vi "ASI_serialRelativeMove setpoint.vi"(2 "VISA resource name":refnum<visa-resource-name>="COM7", 3 "error in (no error)":errorcluster, 4 "setpoint":i32, 5 "Axis":string) -> (0 "error out":errorcluster)   [LabVIEW 2015]
doc: "Establishes connection with configured port (default = COM1).\nSends command MOVE X=x Y=y where x and y are integers denoting 10ths of a micron.\nSub-VI SerialWaitForStatusN.vi polls controller with STATUS command until 'N' (not busy) status is returned, or until a configured maximum number of unsuccessful tries (default = 400).\nDisconnects from configured port."
uses:
  <vilib>/Instr/_visa.llb/VISA Flush IO Buffer Mask.ctl
  Instance           1 20Saved   SerialMoveXY .vi
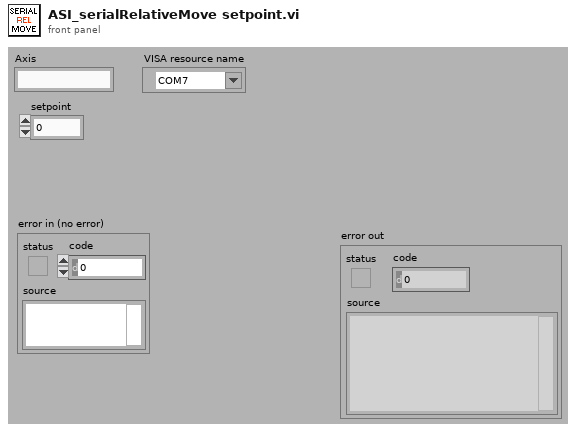
[diagram p1: front panel]
types:
  T1 = typedef "VISA Flush IO Buffer Mask.ctl" = u16
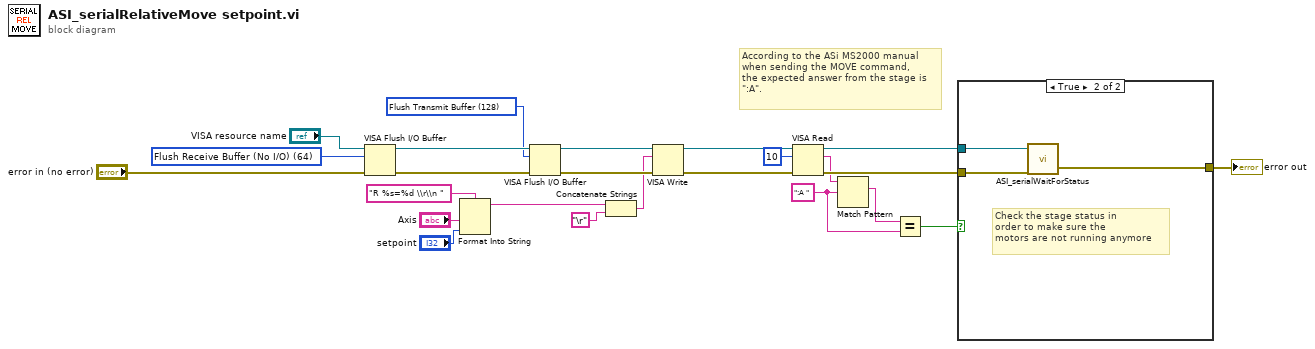
[diagram p0: block diagram]
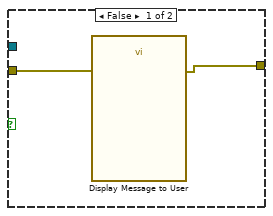
[diagram p2: hidden frame]
diagram:
  w12 = T1 128 items=["Flush Receive Buffer"=16, "Write Transmit Buffer to Device"=32, "Flush Receive Buffer (No I/O)"=64, "Flush Transmit Buffer"=128] ("Mask")
  w15 = T1 64 items=["Flush Receive Buffer"=16, "Write Transmit Buffer to Device"=32, "Flush Receive Buffer (No I/O)"=64, "Flush Transmit Buffer"=128] ("Mask")
  w1 = ":A " ("y")
  # "According to the ASi MS2000 manual\nwhen sending the MOVE command, \nthe expected answer from the stage is\n\":A\"."
  n1 = VISA Flush I/O Buffer(VISA resource name="VISA resource name", mask (16)=w15, error in (no error)="error in (no error)") -> (VISA resource name out=w13:refnum<visa-resource-name>, error out=w14:errorcluster)
  n2 = Format Into String "Format Into String"(format string="R %s=%d \\r\\n ", "Axis", "setpoint") -> (resulting string=w6:string)  [unwired: 2 in, 1 out]
  n3 = VISA Flush I/O Buffer(VISA resource name=w13, mask (16)=w12, error in (no error)=w14) -> (VISA resource name out=w10:refnum<visa-resource-name>, error out=w11:errorcluster)
  n4 = Concatenate Strings(w6, "\r") -> (w4:string)
  n5 = VISA Write(VISA resource name=w10, write buffer=w4, error in (no error)=w11) -> (VISA resource name out=w22:refnum<visa-resource-name>, error out=w7:errorcluster)  [unwired: 1 out]
  n6 = VISA Read(VISA resource name=w22, byte count=u32 10, error in (no error)=w7) -> (VISA resource name out=w19:refnum<visa-resource-name>, read buffer=w3:string, error out=w18:errorcluster)  [unwired: 1 out]
  n7 = Match Pattern(string=w3, regular expression=w1) -> (match substring=w2:string)  [unwired: 1 in, 3 out]
  n8 = Equal?(x=w2, y=w1) -> (x = y?=w20:bool)
  n9 = case shown="True" w20 {
    tunnel: w19 -> [_ w27]
    tunnel: w18 -> [w26 w29]
    tunnel: [w25 w28] -> w8
    frame False {
      n10 = call "Display Message to User"("error in (no error)"=w26) -> ("error out"=w25:errorcluster)  [unwired: 9 in, 1 out]
    }
    frame True {
      # "Check the stage status in\norder to make sure the \nmotors are not running anymore"
      n11 = call "ASI_serialWaitForStatus.vi"("error in"=w29, "VISA resource name"=w27) -> ("error out"=w28:errorcluster)  [unwired: 1 in]
    }
  }
  "error out" <- w8
